vi "Begin.vi"(8 "error in (no error)":errorcluster, 9 "count(-1)":i8=-1, 10 "PreScale":u8, 11 "PCA in":refnum<class "PCA.lvclass">) -> (0 "error out":errorcluster, 2 "Boolean":bool, 3 "PCA out":refnum<class "PCA.lvclass">)   [LabVIEW 2022 SP3, in "PCA9685.lvlib" / "PCA.lvclass"]
uses:
  PCA.lvclass
  PCA.lvclass/PCA.ctl
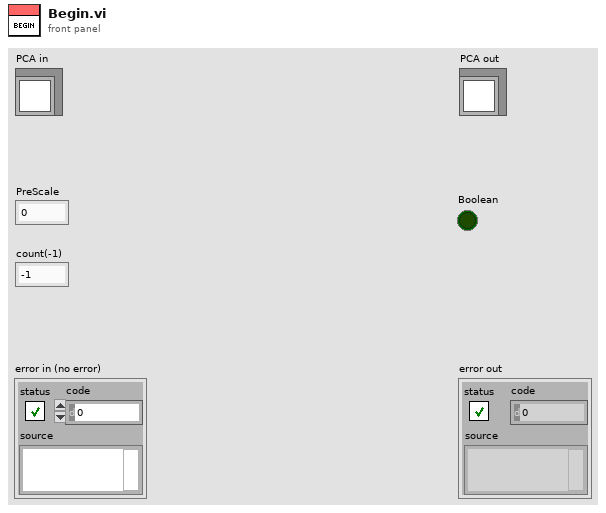
[diagram p1: front panel]
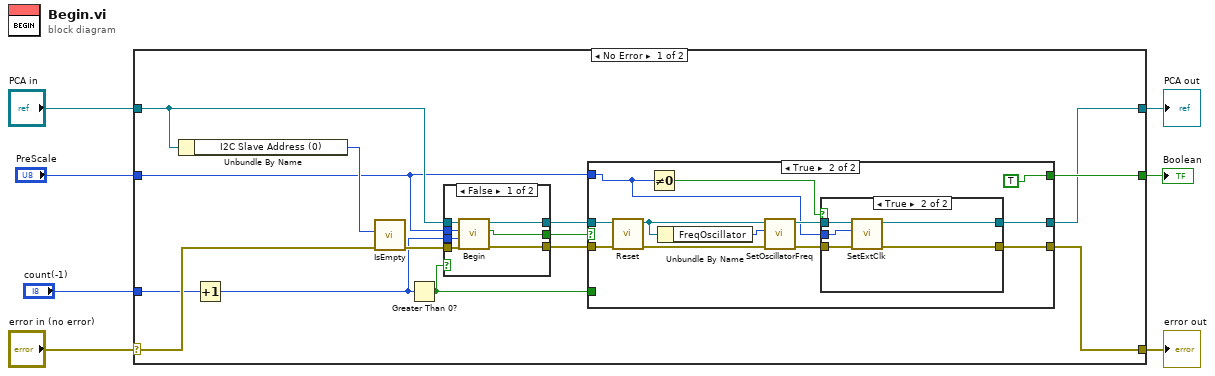
[diagram p0: block diagram]
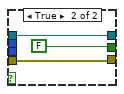
[diagram p2: hidden frame]
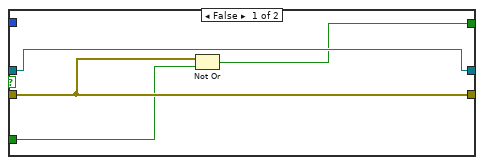
[diagram p3: hidden frame]
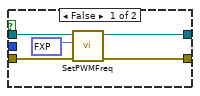
[diagram p4: hidden frame]
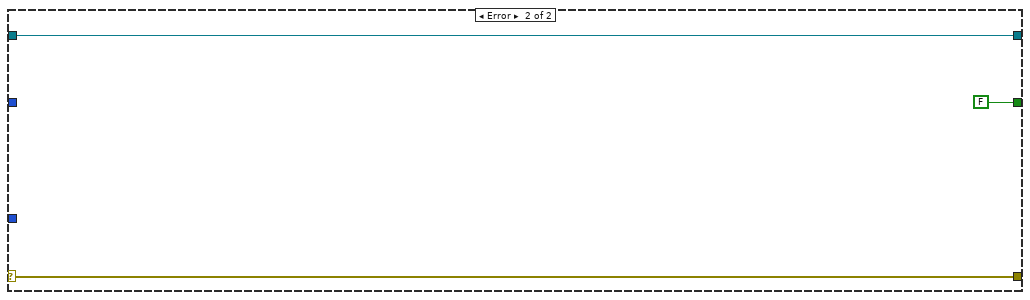
[diagram p5: hidden frame]
diagram:
  n1 = case shown="No Error" "error in (no error)" {
    selector: "error in (no error)" -> [w20 w60]
    tunnel: [w13 w60] -> w6
    tunnel: [w8 w59] -> w4
    tunnel: "PCA in" -> [w19 w59]
    tunnel: "PreScale" -> [w12 _]
    tunnel: [w16 FALSE] -> w2
    tunnel: "count(-1)" -> [w11 _]
    frame No Error {
      n2 = Unbundle By Name(w19) -> ("I2C Slave Address (0)"=w21:u16)
      n3 = Increment(x=w11) -> (x+1=w10:i8)
      n4 = call "IsEmpty.vi"("error in"=w20, "number"=w21) -> ("error out"=w18:errorcluster)  [unwired: 9 in]
      n5 = Greater Than 0?(x=w10) -> (x > 0?=w9:bool)
      n6 = case shown="False" w9 {
        tunnel: w19 -> [w28 w31]
        tunnel: w18 -> [w27 w30]
        tunnel: [w26 FALSE] -> w17
        tunnel: [w25 w30] -> w15
        tunnel: [w24 w31] -> w14
        tunnel: w12 -> [w23 _]
        tunnel: w10 -> [w22 _]
        frame False {
          n7 = call "Begin.vi"("error in (no error)"=w27, "count(-1)"=w22, "PreScale"=w23, "PCA in"=w28) -> ("error out"=w25:errorcluster, "Boolean"=w26:bool, "PCA out"=w24:refnum<class "PCA.lvclass">)  [unwired: 5 in]
        }
        frame True {
        }
      }
      n8 = case shown="True" w17 {
        tunnel: [w32 TRUE] -> w16
        tunnel: w15 -> [w34 w46]
        tunnel: [w34 w37] -> w13
        tunnel: w14 -> [w35 w45]
        tunnel: w12 -> [_ w38]
        tunnel: w9 -> [w33 _]
        tunnel: [w35 w36] -> w8
        frame False {
          n9 = Not Or(1:w33, 2:w34) -> (0:w32:bool)
        }
        frame True {
          n10 = call "Reset.vi"("error in (no error)"=w46, "PCA in"=w45) -> ("error out"=w44:errorcluster, "PCA out"=w42:refnum<class "PCA.lvclass">)  [unwired: 8 in]
          n11 = Not Equal To 0?(x=w38) -> (x != 0?=w41:bool)
          n12 = Unbundle By Name(w42) -> ("FreqOscillator"=w43:u32)
          n13 = call "SetOscillatorFreq.vi"("error in (no error)"=w44, "_oscillator_freq"=w43, "PCA in"=w42) -> ("error out"=w40:errorcluster, "PCA out"=w39:refnum<class "PCA.lvclass">)  [unwired: 7 in]
          n14 = case shown="True" w41 {
            tunnel: w40 -> [w52 w57]
            tunnel: w39 -> [w51 w56]
            tunnel: w38 -> [_ w53]
            tunnel: [w50 w55] -> w37
            tunnel: [w49 w54] -> w36
            frame False {
              n15 = call "SetPWMFreq.vi"("error in (no error)"=w52, "Freq"=fxp<+/-,64,32> 1000.0, "PCA in"=w51) -> ("error out"=w50:errorcluster, "PCA out"=w49:refnum<class "PCA.lvclass">)  [unwired: 7 in]
            }
            frame True {
              n16 = call "SetExtClk.vi"("error in (no error)"=w57, "PreScale"=w53, "PCA in"=w56) -> ("error out"=w55:errorcluster, "PCA out"=w54:refnum<class "PCA.lvclass">)  [unwired: 7 in]
            }
          }
        }
      }
    }
    frame Error {
    }
  }
  "error out" <- w6
  "PCA out" <- w4
  "Boolean" <- w2
